vi "wavelength spectrum to frequency w interpolation.vi"(11 "Input spectrum (nm)":T1) -> (1 "interpix spacing after interpolation (Hz)":dbl, 2 "interpolated amplitudes":dbl[](array[numeric]), 3 "spectrum and interpolated spectrum":cluster{"Ramp Pattern":dbl[], "yi":dbl[]}[](array[cluster]))   [LabVIEW 2013]
uses:
  <vilib>/Analysis/1siggen.llb/Ramp Pattern by Samples.vi
  <vilib>/gmath/NI_Gmath.lvlib
  <vilib>/Analysis/NI_AALBase.lvlib
panel:
  out "XY Graph 2":cluster{"Ramp Pattern":dbl[], "yi":dbl[]}[](graph)
  out "XY Graph":T1(graph)
  out "error out":errorcluster
  out "error":i32
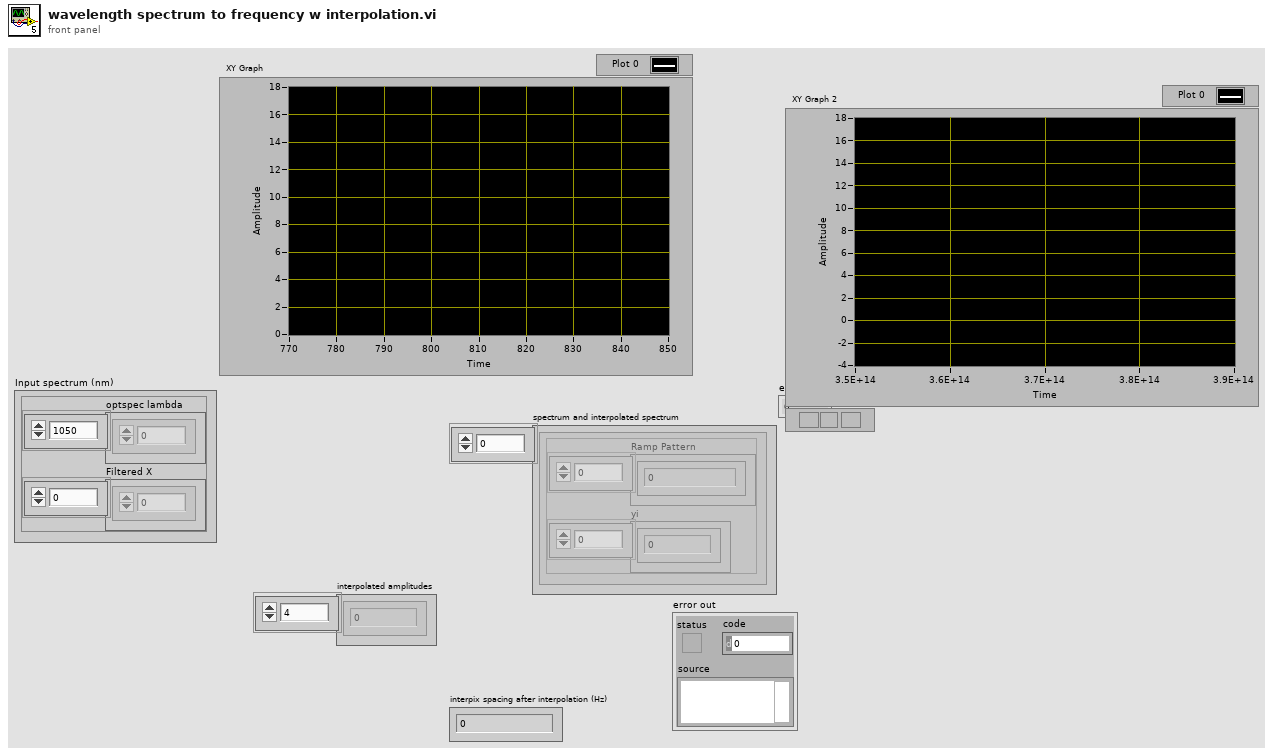
[diagram p1: front panel]
types:
  T1 = cluster{"optspec lambda":dbl[], "Filtered X":dbl[]}
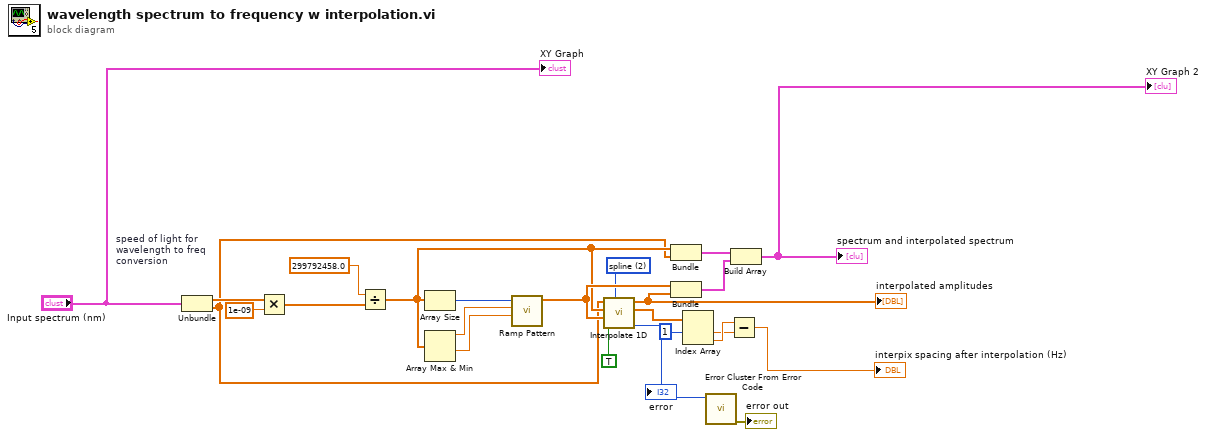
[diagram p0: block diagram]
diagram:
  w1 = 2 items=["nearest", "linear", "spline", "cubic Hermite", "Lagrange"] ("method")
  w7 = 299792458.0  # speed of light for wavelength to freq conversion
  n1 = Unbundle("Input spectrum (nm)") -> ("optspec lambda"=w14:dbl[], "Filtered X"=w11:dbl[])
  n2 = Multiply(x=w14, y=1e-09) -> (x*y=w13:dbl[])
  n3 = Divide(x=w7, y=w13) -> (x/y=w12:dbl[])
  n4 = Array Size(array=w12) -> (size(s)=w8:i32)
  n5 = Array Max & Min(array=w12) -> (max value=w21:dbl, min value=w20:dbl)  [unwired: 2 out]
  n6 = call-poly <vilib>:"Ramp Pattern.vi"("start"=w20, "end"=w21, "samples"=w8) -> ("Ramp Pattern"=w18:dbl[])  [unwired: 7 in, 1 out]
  n7 = call <vilib>:"Interpolate 1D.vi"("method"=w1, "X is monotonic"=TRUE, "xi"=w18, "X"=w12, "Y"=w11) -> ("error"=w5:i32, "xi used"=w16:dbl[], "yi"=w17:dbl[])  [unwired: 4 in]
  "interpolated amplitudes" <- w17
  "error" <- w5
  n8 = Bundle(w12, "Filtered X"=w11) -> (w10:cluster{dbl[], "Filtered X":dbl[]})  [unwired: 1 in]
  n9 = Bundle("Ramp Pattern"=w18, "yi"=w17) -> (w19:cluster{"Ramp Pattern":dbl[], "yi":dbl[]})  [unwired: 1 in]
  n10 = Index Array(array=w16, index #1=1 ("index")) -> (element #1=w23:dbl, element #2=w24:dbl)  [unwired: 1 in]
  n11 = call <vilib>:"Error Cluster From Error Code.vi"("error code (0)"=w5) -> ("error out"=→"error out":errorcluster)  [unwired: 8 in]
  n12 = Subtract(x=w24, y=w23) -> (x-y=→"interpix spacing after interpolation (Hz)":dbl)
  n13 = Build Array(w10, w19) -> (→"spectrum and interpolated spectrum" →"XY Graph 2":cluster{"Ramp Pattern":dbl[], "yi":dbl[]}[])
  "XY Graph" <- "Input spectrum (nm)"
